vi "ATF-Pump-AO Start.vi"(8 "error in":errorcluster, 9 "AO config":T1(array[cluster]), 11 "Refnum in":refnum<k21>) -> (0 "error out":errorcluster, 3 "Refnum out":refnum<k21>)   [LabVIEW 2022 SP3]
doc: "This VI is for start for Analog Output"
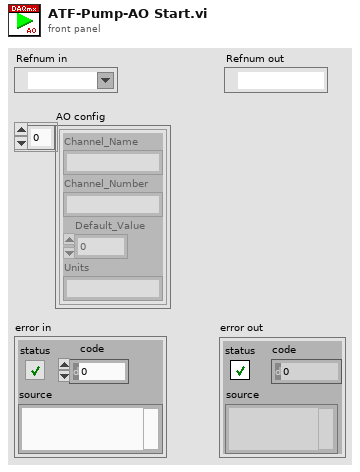
[diagram p1: front panel]
types:
  T1 = cluster{"Channel_Name":string, "Channel_Number":string, "Default_Value":dbl, "Units":string}[]
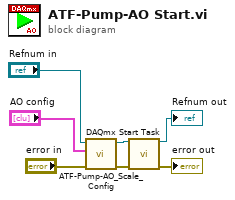
[diagram p0: block diagram]
diagram:
  n1 = call "ATF-Pump-AO_Scale_Config.vi"("error in (no error)"="error in", "AO config"="AO config", "Refnum in"="Refnum in") -> ("error out"=w6:errorcluster, "Refnum out"=w5:refnum<k21>)  [unwired: 7 in]
  n2 = call <vilib>:"DAQmx Start Task.vi"("task/channels in"=w5, "error in"=w6) -> ("task out"=→"Refnum out":refnum<k21>, "error out"=→"error out":errorcluster)  [unwired: 12 in]
